vi "Automated Controllers Test.vi"() -> ()   [LabVIEW 2020, in "Hardware Abstraction App.lvclass"]
uses:
  Hardware Abstraction App/Hardware Abstraction App.lvclass
  Devices/PLC/PLC.lvclass
  C:/Users/fflores/Documents/GitHub Projects/OOP-Concepts-in-LabVIEW/Relations Between Objects/Interface Implemetation/Devices/AutomatedController/AutomatedController.lvclass
  Devices/OPC/OPC.lvclass
  Devices/cRIO/cRIO.lvclass
  ESP8266/ESP8266.lvclass
  Devices/Arduino/Arduino.lvclass
  Wi-Fi Shield/Wi-Fi Shield.lvclass
  C:/Users/fflores/Documents/GitHub Projects/OOP-Concepts-in-LabVIEW/Relations Between Objects/Interface Implemetation/Arduino Shield/Arduino Shield.lvclass
  Devices/Arduino/Arduino.lvclass/Arduino.ctl
  Arduino Shield/Arduino Shield.lvclass
  Devices/AutomatedController/AutomatedController.lvclass
panel:
  in  "Stop Button":bool
  in  "Dispositivo":i32(listbox)=3
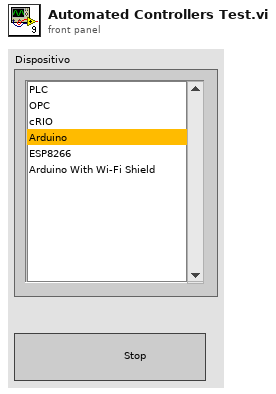
[diagram p1: front panel]
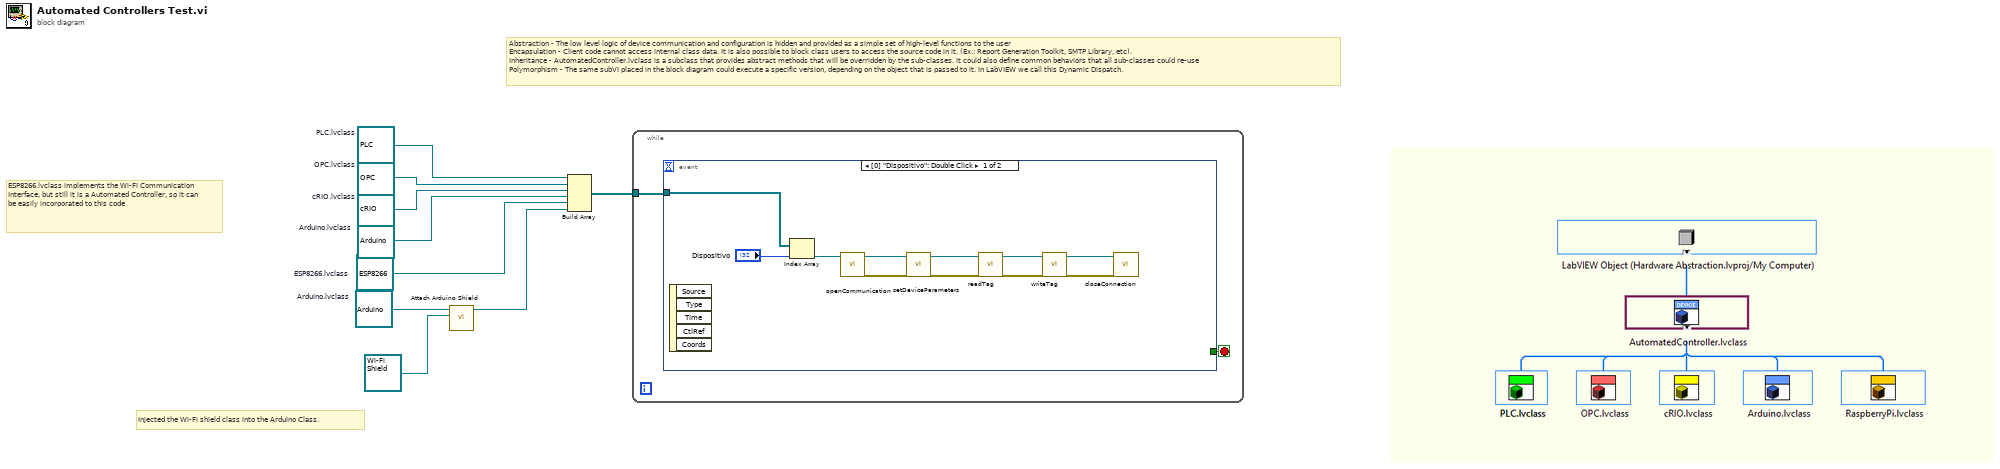
[diagram p0: block diagram]
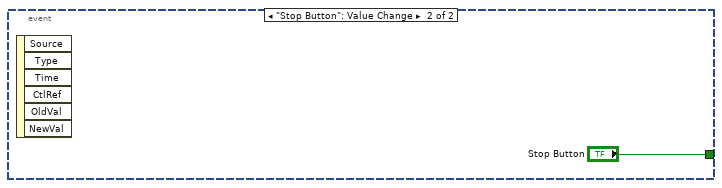
[diagram p2: hidden frame]
diagram:
  w3 = refnum<class "Arduino.lvclass"> refnum  # Arduino.lvclass
  w4 = refnum<class "ESP8266.lvclass"> refnum  # ESP8266.lvclass
  w6 = refnum<class "Arduino.lvclass"> refnum  # Arduino.lvclass
  w7 = refnum<class "cRIO.lvclass"> refnum  # cRIO.lvclass
  w8 = refnum<class "OPC.lvclass"> refnum  # OPC.lvclass
  w9 = refnum<class "PLC.lvclass"> refnum  # PLC.lvclass
  # "Injected the Wi-Fi shield class into the Arduino Class."
  # "ESP8266.lvclass implements the Wi-FI Communication Interface, but still it is a Automated Controller, so it can be easily incorporated to this code"
  # "Abstraction - The low level logic of device communication and configuration is hidden and provided as a simple set of high-level functions to the user\nEncapsulation - Client code cannot access internal class data. It is also possible to block class users to access the source code in it. (Ex.: Report Generation Toolkit, SMTP Library, etc).\nInheritance - AutomatedController.lvclass is a subclass that provides abstract methods that will be overridden by the sub-classes. it could also define common behaviors that all sub-classes could re-use\nPolymorphism - The same subVI placed in the block diagram could execute a specific version, depending on the object that is passed to it. In LabVIEW we call this Dynamic Dispatch."
  n1 = call "Attach Arduino Shield.vi"("Arduino Shield"=refnum<class "Wi-Fi Shield.lvclass"> refnum ("Wi-Fi Shield.lvclass"), "Arduino in"=w3) -> ("Arduino out"=w2:refnum<class "Arduino.lvclass">)  [unwired: 8 in, 1 out]
  n2 = Build Array(w9, w8, w7, w6, w4, w2) -> (w5:refnum<class "AutomatedController.lvclass">[])
  n3 = while {
    tunnel: w5 -> [w10]
    stop <- w11 stop-if-true
    n4 = event shown="[0] \"Dispositivo\": Double Click" {
      selector: _ -> [_ _]
      dyn-events: _ -> [_ _]
      timeout: _ -> [_ _]
      tunnel: [_ "Stop Button"] -> w11
      tunnel: w10 -> [w15 _]
      event "Dispositivo": Double Click {
        n5 = event-data() -> ()  [unwired: 1 in, 5 out]
        n6 = Index Array(array=w15, index="Dispositivo") -> (element=w13:refnum<class "AutomatedController.lvclass">)
        n7 = call-dynamic "openCommunication.vi"("AutomatedController in"=w13) -> ("error out"=w21:errorcluster, "AutomatedController out"=w22:refnum<class "AutomatedController.lvclass">)  [unwired: 9 in]
        n8 = call-dynamic "setDeviceParameters.vi"("error in (no error)"=w21, "AutomatedController in"=w22) -> ("error out"=w20:errorcluster, "AutomatedController out"=w12:refnum<class "AutomatedController.lvclass">)  [unwired: 8 in]
        n9 = call-dynamic "readTag.vi"("error in (no error)"=w20, "AutomatedController in"=w12) -> ("error out"=w18:errorcluster, "AutomatedController out"=w19:refnum<class "AutomatedController.lvclass">)  [unwired: 8 in]
        n10 = call-dynamic "writeTag.vi"("error in (no error)"=w18, "AutomatedController in"=w19) -> ("error out"=w16:errorcluster, "AutomatedController out"=w17:refnum<class "AutomatedController.lvclass">)  [unwired: 8 in]
        n11 = call-dynamic "closeConnection.vi"("error in (no error)"=w16, "AutomatedController in"=w17) -> ()  [unwired: 8 in, 2 out]
      }
      event "Stop Button": Value Change {
        n12 = event-data() -> ()  [unwired: 1 in, 6 out]
      }
    }
  }
